vi "GetType.vi"(8 "error in (no error)":errorcluster, 11 "Send Software Resume Trigger [RT] Msg":refnum<class "Send Software Resume Trigger [RT] Msg.lvclass">) -> (0 "error out":errorcluster, 2 "Data Sample":variant, 3 "Send Software Resume Trigger [RT] Msg":refnum<class "Send Software Resume Trigger [RT] Msg.lvclass">)   [LabVIEW 2015, in "CS++Fgen.lvlib" / "Send Software Resume Trigger [RT] Msg.lvclass"]
doc: "This VI delivers a sample of the data type format the message expects."
uses:
  Send Software Resume Trigger [RT] Msg.lvclass
  Send Software Resume Trigger [RT] Msg.lvclass/Send Software Resume Trigger [RT] Msg.ctl
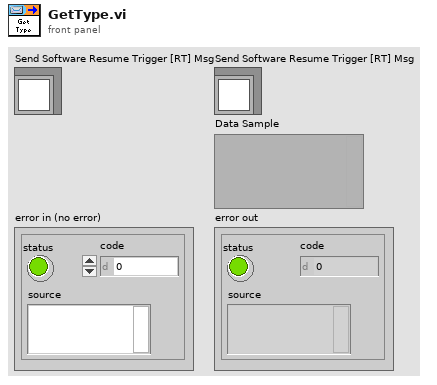
[diagram p1: front panel]
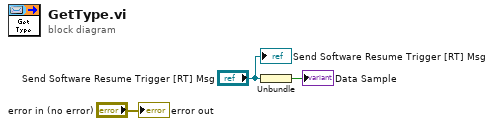
[diagram p0: block diagram]
diagram:
  n1 = Unbundle("Send Software Resume Trigger [RT] Msg") -> (→"Data Sample":bool)
  "error out" <- "error in (no error)"
  "Send Software Resume Trigger [RT] Msg" <- "Send Software Resume Trigger [RT] Msg"
